vi "Get Named Nested Tag Data.vi"(8 "error in (no error)":errorcluster, 10 "Path":cluster{"Tag Name":string, "Index":i32}[](array[cluster]), 11 "Raw Message in":refnum<class "Raw Message.lvclass">) -> (0 "error out":errorcluster, 1 "Tag Data":variant, 2 "Key not found?":bool, 3 "Raw Message out":refnum<class "Raw Message.lvclass">)   [LabVIEW 2020]
uses:
  Raw Message.lvclass
  Raw Message.lvclass/Raw Message.ctl
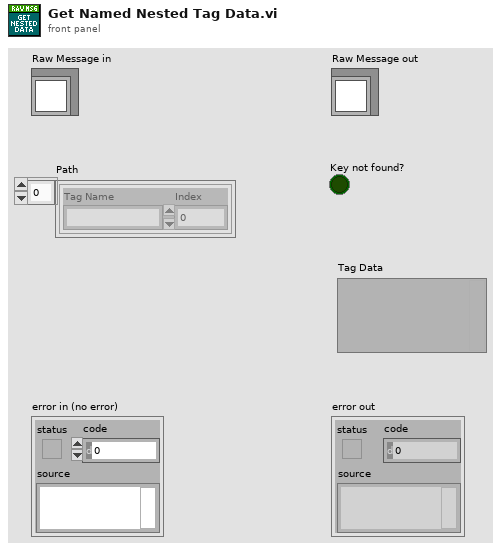
[diagram p1: front panel]
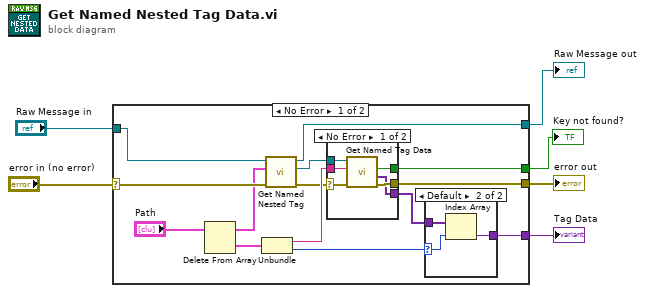
[diagram p0: block diagram]
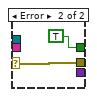
[diagram p3: hidden frame]
diagram:
  n1 = case shown="No Error" "error in (no error)" {
    selector: "error in (no error)" -> [w20 w34]
    tunnel: [w14 w34] -> w5
    tunnel: [w8 w33] -> w3
    tunnel: "Raw Message in" -> [w19 w33]
    tunnel: [w13 _] -> w2
    tunnel: [w11 _] -> w1
    frame No Error {
      n2 = Delete From Array(array="Path") -> (deleted portion=w17:cluster{"Tag Name":string, "Index":i32}, array with subset deleted=w18:cluster{"Tag Name":string, "Index":i32}[])  [unwired: 2 in]
      n3 = Unbundle(w17) -> ("Tag Name"=w16:string, "Index"=w10:i32)
      n4 = call "Get Named Nested Tag.vi"("error in (no error)"=w20, "Path"=w18, "Raw Message in"=w19) -> ("error out"=w15:errorcluster, "Nested Message"=w9:refnum<class "Raw Message.lvclass">, "Raw Message out"=w8:refnum<class "Raw Message.lvclass">)  [unwired: 6 in]
      n5 = case shown="No Error" w15 {
        selector: w15 -> [w28 w31]
        tunnel: w16 -> [w30 _]
        tunnel: w9 -> [w29 _]
        tunnel: [w27 w31] -> w14
        tunnel: [w26 TRUE ("Key not found?")] -> w13
        tunnel: [w25 _] -> w12
        frame No Error {
          n6 = call "Get Named Tag Data.vi"("error in (no error)"=w28, "Tag Name"=w30, "Raw Message in"=w29) -> ("error out"=w27:errorcluster, "Tag Data"=w25:variant[], "Key not found?"=w26:bool)  [unwired: 5 in, 1 out]
        }
        frame Error {
        }
      }
      n7 = case shown="Default" w10 {
        selector: w10 -> [_ w22]
        tunnel: w12 -> [w21 w24]
        tunnel: [w21 w23] -> w11
        frame -1 {
        }
        frame Default {
          n8 = Index Array(array=w24, index=w22) -> (element=w23:variant)
        }
      }
    }
    frame Error {
    }
  }
  "error out" <- w5
  "Raw Message out" <- w3
  "Key not found?" <- w2
  "Tag Data" <- w1
